vi "Layer Scan V2.vi"() -> ()   [LabVIEW 2024]
uses:
  <vilib>/userDefined/High Color/IMAQdx.ctl
  <vilib>/DAQmx/write.llb/DAQmx Write (Analog 2D DBL NChan NSamp).vi
  <vilib>/DAQmx/write.llb/DAQmx Write (Analog 1D DBL NChan 1Samp).vi
  <vilib>/DAQmx/read.llb/DAQmx Read (Analog 1D DBL 1Chan NSamp).vi
  <vilib>/DAQmx/create/channels.llb/DAQmx Create Channel (AO-Voltage-Basic).vi
  <vilib>/DAQmx/miscellaneous.llb/DAQmx Fill In Error Info.vi
  <vilib>/DAQmx/create/channels.llb/DAQmx Create Channel (AI-Voltage-Basic).vi
  <vilib>/DAQmx/configure/timing.llb/DAQmx Timing (Sample Clock).vi
  <vilib>/vision/driver/NI_Vision_Acquisition_Software.lvlib
  <vilib>/measure/NI_MABase.lvlib
panel:
  out "Most recent image filename":string
  in  "Image Name":path
  in  "Image Folder Path":path
  out "most recent Image saved":T1(plugin-control)
  out "Current Data Filename":string
  in  "Data File Name":path
  in  "Folder Path":path
  out "?":dbl
  out "?":dbl
  out "Filename Out":path
  in  "Y desired voltage step(V/100)":dbl=1.0 format="%#_13g"
  in  "X desired voltage step(V/100)":dbl=1.0 format="%#_13g"
  out "Y MIN":dbl
  out "Y MAX":dbl
  out "X MIN":dbl
  out "X MAX":dbl
  out "Waveform Chart":waveform(dbl)(graph)
  out "Waveform Chart 2":waveform(dbl)(graph)
  in  "offset X":dbl format="%0.2p"
  in  "amplitude X":dbl=1.0 format="%0.2p"
  in  "amplitude Y":dbl=1.0 format="%0.2p"
  in  "offset Y":dbl format="%0.2p"
  in  "COMMENCE SCAN":bool
  out "Waveform Graph 2":waveform(dbl)(graph)
  out "Waveform Graph":dbl[](graph)
  # "Mirror angle Signal"
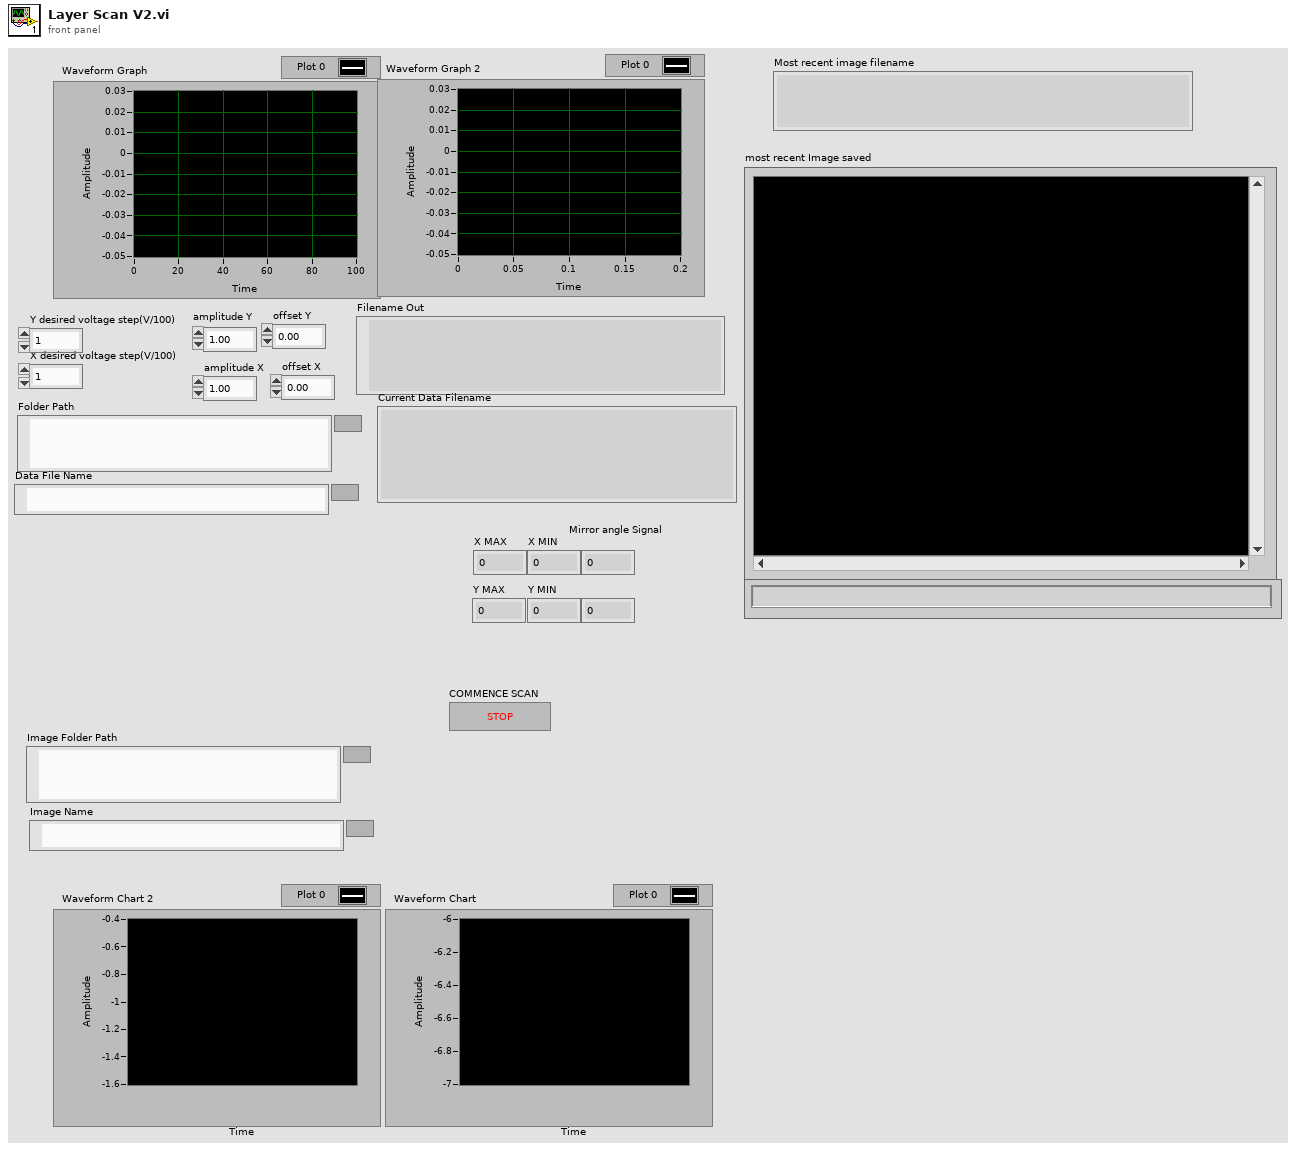
[diagram p1: front panel]
types:
  T1 = typedef "IMAQ Image.ctl" = refnum<image>
  T2 = typedef "IMAQdx.ctl" = refnum<k21>
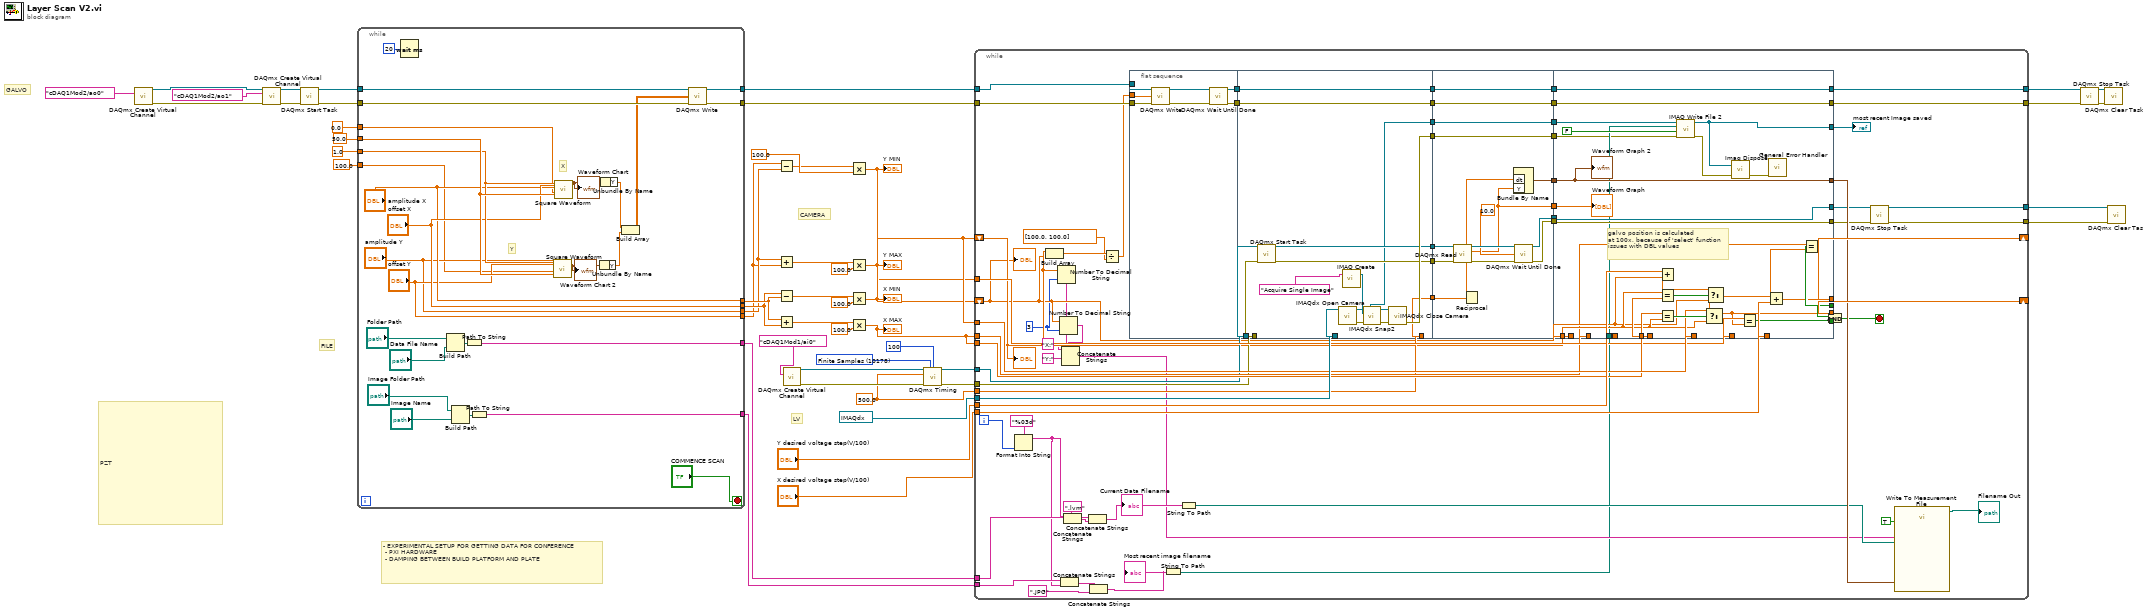
[diagram p0: block diagram]
diagram:
  w13 = 10178 items=["Finite Samples"=10178, "Continuous Samples"=10123, "Hardware Timed Single Point"=12522] ("sample mode")
  w15 = 500.0 ("rate")
  # "- EXPERIMENTAL SETUP FOR GETTING DATA FOR CONFERENCE\n - PXI HARDWARE\n - DAMPING BETWEEN BUILD PLATFORM AND PLATE"
  # "PZT"
  # "FILE"
  # "LV"
  # "GALVO"
  # "CAMERA"
  n1 = call-poly <vilib>:"DAQmx Create Virtual Channel.vi"("physical channels"=tag "cDAQ1Mod2/ao0") -> ("task out"=w48:refnum<k21>, "error out"=w47:errorcluster)  [unwired: 13 in]
  n2 = call-poly <vilib>:"DAQmx Create Virtual Channel.vi"("task in"=w48, "physical channels"=tag "cDAQ1Mod2/ao1", "error in"=w47) -> ("task out"=w44:refnum<k21>, "error out"=w43:errorcluster)  [unwired: 11 in]
  n3 = call <vilib>:"DAQmx Start Task.vi"("task/channels in"=w44, "error in"=w43) -> ("task out"=w42:refnum<k21>, "error out"=w41:errorcluster)  [unwired: 12 in]
  n4 = while {
    tunnel: 50.0 ("duty cycle (%)") -> [w76]
    tunnel: 1.0 ("frequency") -> [w75]
    tunnel: w42 -> [w72]
    tunnel: w41 -> [w71]
    tunnel: [w65] -> w38
    tunnel: [w64] -> w37
    tunnel: ["offset X"] -> w27
    tunnel: ["amplitude X"] -> w28
    tunnel: ["offset Y"] -> w25
    tunnel: ["amplitude Y"] -> w26
    tunnel: 0.0 ("phase") -> [w59]
    tunnel: 100.0 ("phase") -> [w58]
    tunnel: [w54] -> w4
    tunnel: [w50] -> w1
    stop <- "COMMENCE SCAN" stop-if-true
    # "Y"
    # "X"
    n5 = Wait (ms)(milliseconds to wait=u32 20) -> ()  [unwired: 1 out]
    n6 = Build Path(base path="Folder Path", name or relative path="Data File Name") -> (appended path=w55:path)
    n7 = Build Path(base path="Image Folder Path", name or relative path="Image Name") -> (appended path=w53:path)
    n8 = Path To String(path=w55) -> (string=w54:string)
    n9 = Path To String(path=w53) -> (string=w50:string)
    n10 = call <vilib>:"Square Waveform.vi"("duty cycle (%)"=w76, "offset"="offset Y", "phase"=w58, "amplitude"="amplitude Y", "frequency"=w75) -> ("signal out"=w70:waveform(dbl))  [unwired: 5 in, 1 out]
    "Waveform Chart 2" <- w70
    n11 = call <vilib>:"Square Waveform.vi"("duty cycle (%)"=w76, "offset"="offset X", "phase"=w59, "amplitude"="amplitude X", "frequency"=w75) -> ("signal out"=w69:waveform(dbl))  [unwired: 5 in, 1 out]
    "Waveform Chart" <- w69
    n12 = Unbundle By Name(w70) -> ("Y"=w67:dbl[])
    n13 = Unbundle By Name(w69) -> ("Y"=w68:dbl[])
    n14 = Build Array(w68, w67) -> (w66:dbl[][])
    n15 = call-poly <vilib>:"DAQmx Write.vi"("task/channels in"=w72, "data"=w66, "error in"=w71) -> ("task out"=w65:refnum<k21>, "error out"=w64:errorcluster)  [unwired: 10 in, 1 out]
  }
  n16 = Subtract(x=w25, y=w26) -> (x-y=w31:dbl)
  n17 = Add(x=w26, y=w25) -> (x+y=w29:dbl)
  n18 = Subtract(x=w27, y=w28) -> (x-y=w32:dbl)
  n19 = Add(x=w28, y=w27) -> (x+y=w30:dbl)
  n20 = call-poly <vilib>:"DAQmx Create Virtual Channel.vi"("physical channels"=tag "cDAQ1Mod1/ai0") -> ("task out"=w17:refnum<k21>, "error out"=w16:errorcluster)  [unwired: 13 in]
  n21 = Multiply(x=w31, y=100.0) -> (x*y=w7:dbl)
  "Y MIN" <- w7
  n22 = Multiply(x=w29, y=100.0) -> (x*y=w5:dbl)
  "Y MAX" <- w5
  n23 = Multiply(x=w32, y=100.0) -> (x*y=w8:dbl)
  "X MIN" <- w8
  n24 = Multiply(x=w30, y=100.0) -> (x*y=w6:dbl)
  "X MAX" <- w6
  n25 = call-poly <vilib>:"DAQmx Timing.vi"("task/channels in"=w17, "sample mode"=w13, "samples per channel"=100, "rate"=w15, "error in"=w16) -> ("task out"=w12:refnum<k21>, "error out"=w11:errorcluster)  [unwired: 9 in]
  n26 = while {
    tunnel: T2 "cam3" ("Session In") -> [w130]
    tunnel: w38 -> [w129]
    tunnel: w37 -> [w128]
    tunnel: "X desired voltage step(V/100)" -> [w127]
    tunnel: "Y desired voltage step(V/100)" -> [w126]
    tunnel: w8 -> [w125]
    tunnel: w6 -> [w124]
    shift-right: [w123] -> _
    shift-left: w8 -> [w96]
    shift-right: [w122] -> _
    shift-left: w7 -> [w95]
    tunnel: w5 -> [w116]
    tunnel: w6 -> [w115]
    tunnel: [w114] -> w19
    tunnel: [w113] -> w18
    tunnel: w15 -> [w112]
    tunnel: w12 -> [w109]
    tunnel: w11 -> [w108]
    tunnel: [w107] -> w10
    tunnel: [w106] -> w9
    tunnel: w4 -> [w102]
    tunnel: w1 -> [w81]
    i -> [w83]
    stop <- w97 stop-if-true
    w94 = i16 3 ("width (-)")
    n27 = Format Into String(format string="%03d", w83) -> (resulting string=w80:string)  [unwired: 2 in, 1 out]
    n28 = Build Array(w96, w95) -> (w121:dbl[])
    n29 = Number To Decimal String(number=w96, width (-)=w94) -> (decimal integer string=w92:string)
    n30 = Number To Decimal String(number=w95, width (-)=w94) -> (decimal integer string=w90:string)
    n31 = Concatenate Strings(w81, w80) -> (w79:string)
    n32 = Concatenate Strings("X:", w92, "Y:", w90) -> (w89:string)
    n33 = Concatenate Strings(w80, ".lvm") -> (w103:string)
    n34 = Concatenate Strings(w102, w103) -> (w101:string)
    "Current Data Filename" <- w101
    n35 = Concatenate Strings(w79, ".JPG" ("string")) -> (w77:string)
    "Most recent image filename" <- w77
    n36 = Divide(x=w121, y=dbl[] [100.0, 100.0]) -> (x/y=w105:dbl[])
    n37 = flat-sequence {
      tunnel: [w149] -> w144
      tunnel: [w148] -> w143
      tunnel: w129 -> [w147]
      tunnel: w128 -> [w146]
      tunnel: w105 -> [w145]
      tunnel: w130 -> [w161]
      tunnel: w144 -> [w160]
      tunnel: w143 -> [w159]
      tunnel: [w160] -> w142
      tunnel: [w159] -> w141
      tunnel: [w158] -> w140
      tunnel: [w156] -> w139
      tunnel: [w155] -> w138
      tunnel: [w157] -> w137
      tunnel: w112 -> [w157]
      tunnel: w109 -> [w154]
      tunnel: w108 -> [w153]
      tunnel: [w152] -> w87
      tunnel: w142 -> [w182]
      tunnel: w141 -> [w181]
      tunnel: w140 -> [w168]
      tunnel: w139 -> [w177]
      tunnel: w138 -> [w176]
      tunnel: [w182] -> w136
      tunnel: [w181] -> w135
      tunnel: w137 -> [w174]
      tunnel: [w173] -> w134
      tunnel: [w172] -> w133
      tunnel: [w171] -> w132
      tunnel: [w170] -> w131
      tunnel: [w169] -> w88
      tunnel: w87 -> [w169]
      tunnel: [w168] -> w84
      tunnel: [w211] -> w113
      tunnel: [w212] -> w114
      tunnel: w136 -> [w212]
      tunnel: w135 -> [w211]
      tunnel: w134 -> [w196]
      tunnel: w133 -> [w210]
      tunnel: w132 -> [w193]
      tunnel: w131 -> [w192]
      tunnel: w127 -> [w205]
      tunnel: w126 -> [w204]
      tunnel: w125 -> [w203]
      tunnel: w124 -> [w202]
      tunnel: w124 -> [w201]
      tunnel: [w190] -> w123
      tunnel: [w191] -> w122
      tunnel: w96 -> [w200]
      tunnel: w95 -> [w199]
      tunnel: [w198] -> w120
      tunnel: [w197] -> w119
      tunnel: [w196] -> w118
      tunnel: w116 -> [w195]
      tunnel: w115 -> [w194]
      tunnel: [w193] -> w111
      tunnel: [w192] -> w110
      tunnel: w88 -> [w189]
      tunnel: w86 -> [w187]
      tunnel: [w183] -> w85
      tunnel: w84 -> [w185]
      frame #0 {
        n38 = call-poly <vilib>:"DAQmx Write.vi"("task/channels in"=w147, "data"=w145, "error in"=w146) -> ("task out"=w151:refnum<k21>, "error out"=w150:errorcluster)  [unwired: 10 in, 1 out]
        n39 = call <vilib>:"DAQmx Wait Until Done.vi"("task/channels in"=w151, "error in"=w150) -> ("task out"=w149:refnum<k21>, "error out"=w148:errorcluster)  [unwired: 12 in]
      }
      frame #1 {
        n40 = call <vilib>:"DAQmx Start Task.vi"("task/channels in"=w154, "error in"=w153) -> ("task out"=w156:refnum<k21>, "error out"=w155:errorcluster)  [unwired: 12 in]
        n41 = call <vilib>:"IMAQdx Open Camera.vi"("Session In"=w161) -> ("error out"=w166:errorcluster, "Session Out"=w164:T2)  [unwired: 2 in, 7 out]
        n42 = call "IMAQ Create"("Image Name"="Acquire Single Image") -> ("New Image"=w167:T1)  [unwired: 3 in, 2 out]
        n43 = call <vilib>:"IMAQdx Snap2.vi"("error in"=w166, "Image In"=w167, "Session In"=w164) -> ("error out"=w165:errorcluster, "Image Out"=w152:T1, "Session Out"=w163:T2)  [unwired: 6 in]
        n44 = call <vilib>:"IMAQdx Close Camera.vi"("error in"=w165, "Session In"=w163) -> ("error out"=w158:errorcluster)  [unwired: 9 out]
      }
      frame #2 {
        n45 = call-poly <vilib>:"DAQmx Read.vi"("task/channels in"=w177, "error in"=w176) -> ("task out"=w180:refnum<k21>, "data"=w172:dbl[], "error out"=w179:errorcluster)  [unwired: 11 in]
        n46 = Reciprocal(x=w174) -> (1/x=w175:dbl)
        n47 = Bundle By Name("dt"=w175, "Y"=w172) -> (w173:waveform(dbl))  [unwired: 1 in]
        n48 = call <vilib>:"DAQmx Wait Until Done.vi"("task/channels in"=w180, "timeout (sec)"=10.0, "error in"=w179) -> ("task out"=w171:refnum<k21>, "error out"=w170:errorcluster)  [unwired: 11 in]
      }
      frame #3 {
        # "galvo position is calculated\nat 100x, because of 'select' function\nissues with DBL values"
        n49 = Add(x=w204, y=w199) -> (x+y=w207:dbl)
        n50 = Equal?(x=w200, y=w201) -> (x = y?=w208:bool)
        n51 = Equal?(x=w202, y=w200) -> (x = y?=w209:bool)
        n52 = call-poly "IMAQ Write File 2"("error in (no error)"=w185, "Compress? (N)"=FALSE, "File Path"=w187, "Image"=w189) -> ("error out"=w184:errorcluster, "Image Out (duplicate)"=w183:T1)  [unwired: 6 in]
        n53 = Select(t=w203, s=w209, f=w200) -> (s? t:f=w206:dbl)
        n54 = Select(t=w207, s=w208, f=w199) -> (s? t:f=w191:dbl)
        n55 = call "Imaq Dispose"("Image"=w183, "error in (no error)"=w184) -> ("error out"=w186:errorcluster)  [unwired: 4 in]
        n56 = Equal?(x=w195, y=w191) -> (x = y?=w198:bool)
        n57 = Add(x=w206, y=w205) -> (x+y=w190:dbl)
        n58 = call <vilib>:"General Error Handler.vi"("error in (no error)"=w186) -> ()  [unwired: 2 in, 13 out]
        n59 = Equal?(x=w194, y=w190) -> (x = y?=w197:bool)
        "Waveform Graph 2" <- w196
        "Waveform Graph" <- w210
      }
    }
    n60 = String To Path(string=w77) -> (path=w86:path)
    n61 = String To Path(string=w101) -> (path=w100:path)
    n62 = And(x=w119, y=w120) -> (x .and. y?=w97:bool)
    n63 = call <vilib>:"DAQmx Stop Task.vi"("task/channels in"=w111, "error in"=w110) -> ("task out"=w107:refnum<k21>, "error out"=w106:errorcluster)  [unwired: 12 in]
    n64 = call "Write To Measurement File"("Signals"=w118, "Enable"=TRUE, "Filename"=w100, "Comment"=w89) -> ("Filename Out"=→"Filename Out":path)  [unwired: 13 in, 2 out]
    "?" <- w95
    "?" <- w96
    "most recent Image saved" <- w85
  }
  n65 = call <vilib>:"DAQmx Stop Task.vi"("task/channels in"=w19, "error in"=w18) -> ("task out"=w21:refnum<k21>, "error out"=w20:errorcluster)  [unwired: 12 in]
  n66 = call <vilib>:"DAQmx Clear Task.vi"("task in"=w21, "error in"=w20) -> ()  [unwired: 13 in, 1 out]
  n67 = call <vilib>:"DAQmx Clear Task.vi"("task in"=w10, "error in"=w9) -> ()  [unwired: 13 in, 1 out]
